vi "Pre Launch Init.vi"(11 "ForecastData in":refnum<class "ForecastData.lvclass">) -> (0 "error out":errorcluster, 3 "ForecastData out":refnum<class "ForecastData.lvclass">)   [LabVIEW 2018, in "ForecastData Actor.lvlib" / "ForecastData.lvclass"]
doc: "(<B>Filename</B>: Actor Framework.lvlib:Actor.lvclass:Pre Launch Init.vi)\n\nDefines behavior that occurs after the Launch Nested Actor method is invoked but before the actor's Actor Core method begins running.\n\nBy default, this method does nothing. A descendant class may override it to define behavior."
uses:
  ForecastData.lvclass
  C:/Users/Administrator/Desktop/2018LabVIEW EMS/EMS Generic Actor/EMS Generic/EMS Generic.lvclass
  C:/Users/Administrator/Desktop/2018LabVIEW EMS/IED Actors/Device DDS Communications Framework/Device DDS Communications/Device DDS Communications.lvclass
  Device DDS Communications Framework/Device DDS Communications/Device DDS Communications.lvclass/Device DDS Communications.ctl
  <vilib>/ORNL/CSEISMIC DDS/CSEISMIC DDS Base/CSEISMIC DDS.lvclass/CSEISMIC DDS.ctl
  <vilib>/ORNL/CSEISMIC DDS/CSEISMIC DDS Base/Accessors/Write DDS Reference.vi
  <vilib>/ORNL/CSEISMIC DDS/DDS Writer/DDS Writer.lvclass
  C:/Program Files (x86)/National Instruments/LabVIEW 2018/vi.lib/ORNL/CSEISMIC DDS/CSEISMIC DDS Base/CSEISMIC DDS.lvclass
  <vilib>/ORNL/CSEISMIC DDS/CSEISMIC DDS Base/Error Handler.vi
  Device DDS Communications Framework/Device DDS Communications/Device DDS Communications.lvclass
  EMS Generic Actor/EMS Generic/EMS Generic.lvclass
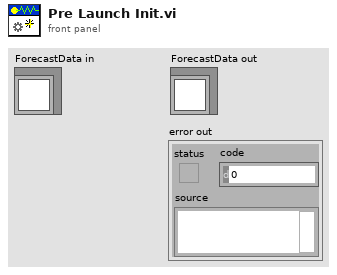
[diagram p1: front panel]
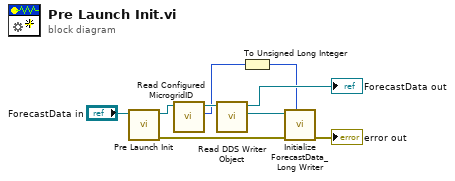
[diagram p0: block diagram]
diagram:
  n1 = call-parent "Pre Launch Init.vi"("Device DDS Communications in"="ForecastData in") -> ("error out"=w3:errorcluster, "Device DDS Communications out"=w6:refnum<class "ForecastData.lvclass">)  [unwired: 9 in]
  n2 = call "Read Configured MicrogridID.vi"("EMS Generic in"=w6) -> ("Microgrid ID"=w7:u8, "EMS Generic out"=w8:refnum<class "ForecastData.lvclass">)  [unwired: 8 in, 1 out]
  n3 = call "Read DDS Writer Object.vi"("Device DDS Communications in"=w8) -> ("DDS Writer Object"=w4:refnum<class "DDS Writer.lvclass">, "Device DDS Communications out"=→"ForecastData out":refnum<class "ForecastData.lvclass">)  [unwired: 9 in]
  n4 = To Unsigned Long Integer(number=w7) -> (unsigned 32bit integer=w1:u32)
  n5 = call <vilib>:"Initialize ForecastData_Long Writer.vi"("MicrogridID"=w1, "error in"=w3, "DDS Writer in"=w4) -> ("error out"=→"error out":errorcluster)  [unwired: 7 in, 1 out]
